vi "Start Scan.vi"(8 "error in (no error)":errorcluster, 10 "Init work":bool, 11 "Keithley 622x2182 Driver in":refnum<class "Keithley 622x2182 Driver.lvclass">) -> (0 "error out":errorcluster, 3 "Keithley 622x2182 Driver out":refnum<class "Keithley 622x2182 Driver.lvclass">)   [LabVIEW 2021, in "Keithley 622x2182 Driver.lvclass"]
uses:
  Keithley 622x2182 Driver.lvclass
  C:/GitHub/NHMFL_Core/Libraries/Instruments/VISA Instrument/VISA Instrument.lvclass
  VISA Instrument/VISA Instrument.lvclass/VISA Instrument.ctl
  VISA Instrument/Read VISA resource.vi
  VISA Instrument/Write VISA resource.vi
  Keithley 622x2182 Driver.lvclass/Keithley 622x2182 Driver.ctl
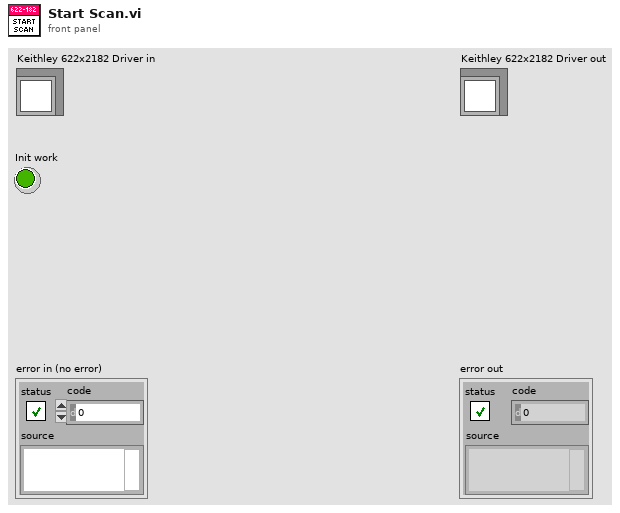
[diagram p1: front panel]
types:
  T1 = enum16{"Delta", "Diff. conductance", "Pulse delta sweep"}
  T2 = typedef "Stepper Config.ctl" = cluster{"Start":dbl, "End":dbl, "Step":dbl, "Delta":dbl, "Scan shape":enum16{"Sawtooth", "Triangular"}, "Append measurements":string[], "Pulse width":dbl, "Pulse interval":dbl, "Scan mode":enum16{"Delta", "Diff. conductance", "Pulse delta sweep"}}
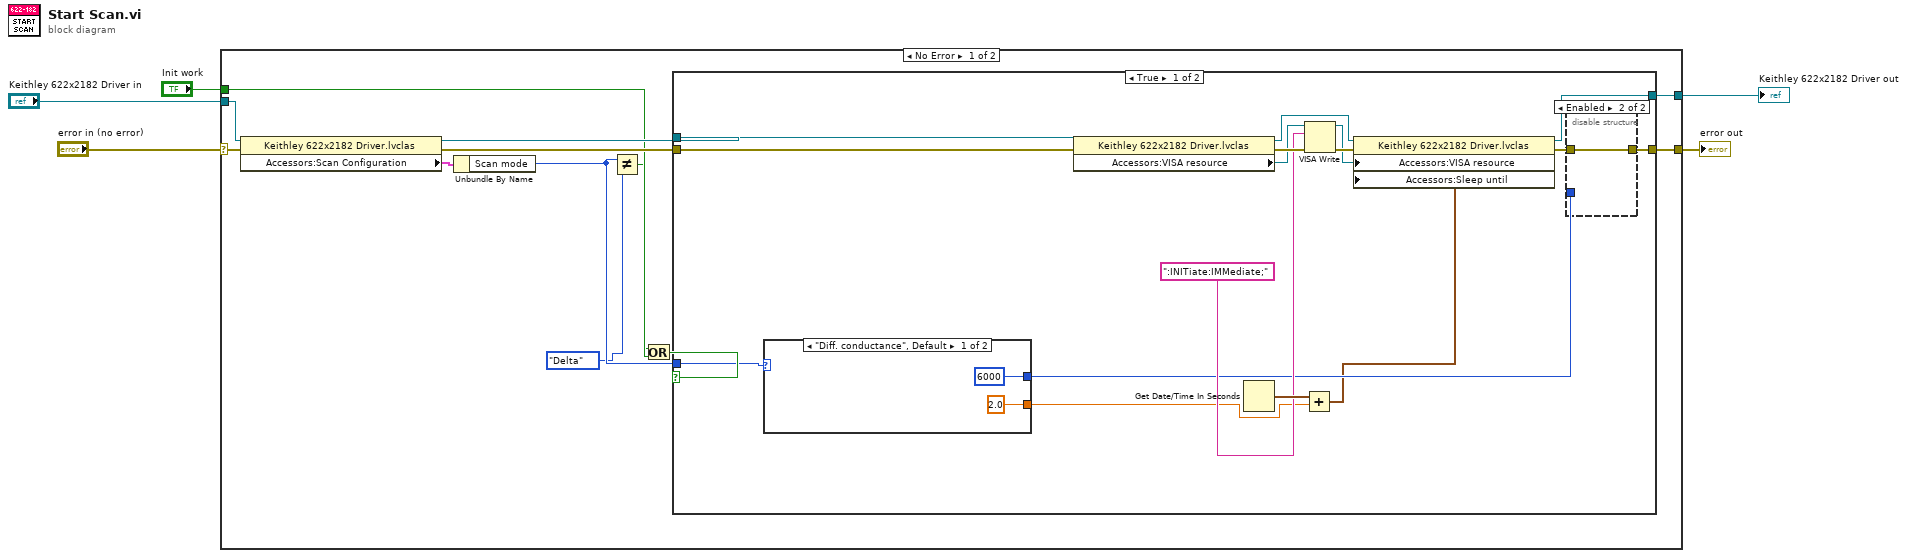
[diagram p0: block diagram]
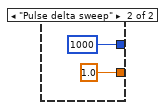
[diagram p2: hidden frame]
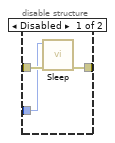
[diagram p3: hidden frame]
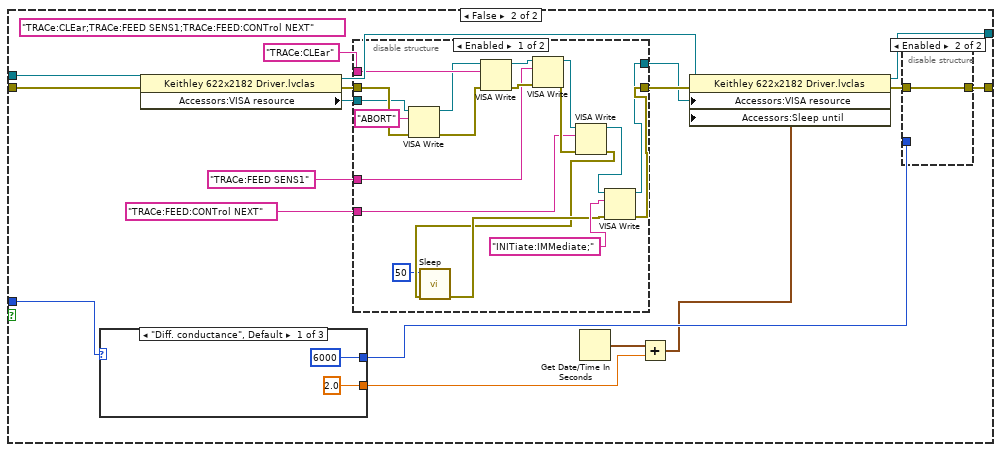
[diagram p4: hidden frame]
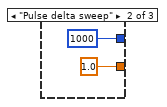
[diagram p6: hidden frame]
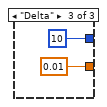
[diagram p7: hidden frame]
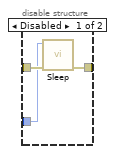
[diagram p8: hidden frame]
diagram:
  n1 = case shown="No Error" "error in (no error)" {
    selector: "error in (no error)" -> [w17 w92]
    tunnel: [w15 w92] -> w4
    tunnel: [w16 w91] -> w2
    tunnel: "Keithley 622x2182 Driver in" -> [w13 w91]
    tunnel: "Init work" -> [w8 _]
    frame No Error {
      n2 = property class="Keithley 622x2182 Driver.lvclas"(reference=w13, error in=w17) -> (reference out=w12:refnum<class "Keithley 622x2182 Driver.lvclass">, error out=w14:errorcluster, "Accessors:Scan Configuration"=w11:T2)
      n3 = Unbundle By Name(w11) -> ("Scan mode"=w10:T1)
      n4 = Not Equal?(x=w10, y=T1."Delta" ("Scan mode")) -> (x != y?=w7:bool)
      n5 = Or(x=w7, y=w8) -> (x .or. y?=w6:bool)
      n6 = case shown="True" w6 {
        tunnel: [w32 w58] -> w16
        tunnel: [w25 w51] -> w15
        tunnel: w10 -> [w23 w49]
        tunnel: w14 -> [w19 w45]
        tunnel: w12 -> [w18 w44]
        frame True {
          n7 = case shown="\"Diff. conductance\", Default" w23 {
            tunnel: [u32 6000 ("milliseconds to wait") u32 1000 ("milliseconds to wait")] -> w22
            tunnel: [2.0 ("y") 1.0 ("y")] -> w20
            frame "Diff. conductance", Default {
            }
            frame "Pulse delta sweep" {
            }
          }
          n8 = property class="Keithley 622x2182 Driver.lvclas"(reference=w18, error in=w19) -> (reference out=w33:refnum<class "Keithley 622x2182 Driver.lvclass">, error out=w30:errorcluster, "Accessors:VISA resource"=w27:refnum<visa-resource-name>)
          n9 = Get Date/Time In Seconds() -> (seconds since 1Jan1904=w31:timestamp)
          n10 = Add(x=w31, y=w20) -> (x+y=w21:timestamp)
          n11 = VISA Write(VISA resource name=w27, write buffer=":INITiate:IMMediate;", error in (no error)=w30) -> (VISA resource name out=w28:refnum<visa-resource-name>, error out=w29:errorcluster)  [unwired: 1 out]
          n12 = property class="Keithley 622x2182 Driver.lvclas"(reference=w33, error in=w29, "Accessors:VISA resource"=w28, "Accessors:Sleep until"=w21) -> (reference out=w32:refnum<class "Keithley 622x2182 Driver.lvclass">, error out=w24:errorcluster)
          n13 = disable-structure shown="Enabled" {
            disable-tunnel: [w40 w41] -> w25
            disable-tunnel: w24 -> [w39 w41]
            disable-tunnel: w22 -> [w38 _]
            frame Disabled {
              n14 = call "Sleep.vi"("error in"=w39, "milliseconds to wait"=w38) -> ("error out"=w40:errorcluster)  [unwired: 9 in]
            }
            frame Enabled {
            }
          }
        }
        frame False {
          (unwired) "TRACe:CLEar;TRACe:FEED SENS1;TRACe:FEED:CONTrol NEXT" ("write buffer")
          n15 = case shown="\"Diff. conductance\", Default" w49 {
            tunnel: [u32 6000 ("milliseconds to wait") u32 1000 ("milliseconds to wait") u32 10 ("milliseconds to wait")] -> w48
            tunnel: [2.0 ("y") 1.0 ("y") 0.01 ("y")] -> w46
            frame "Diff. conductance", Default {
            }
            frame "Pulse delta sweep" {
            }
            frame "Delta" {
            }
          }
          n16 = property class="Keithley 622x2182 Driver.lvclas"(reference=w44, error in=w45) -> (reference out=w59:refnum<class "Keithley 622x2182 Driver.lvclass">, error out=w56:errorcluster, "Accessors:VISA resource"=w53:refnum<visa-resource-name>)
          n17 = disable-structure shown="Enabled" {
            disable-tunnel: w56 -> [w66 w79]
            disable-tunnel: [w71 w79] -> w55
            disable-tunnel: [w69 w80] -> w54
            disable-tunnel: w53 -> [w64 w80]
            disable-tunnel: "TRACe:CLEar" ("write buffer") -> [w78 _]
            disable-tunnel: "TRACe:FEED SENS1" ("write buffer") -> [w75 _]
            disable-tunnel: "TRACe:FEED:CONTrol NEXT" ("write buffer") -> [w72 _]
            frame Enabled {
              n18 = VISA Write(VISA resource name=w64, write buffer="ABORT", error in (no error)=w66) -> (VISA resource name out=w65:refnum<visa-resource-name>, error out=w67:errorcluster)  [unwired: 1 out]
              n19 = VISA Write(VISA resource name=w65, write buffer=w78, error in (no error)=w67) -> (VISA resource name out=w76:refnum<visa-resource-name>, error out=w77:errorcluster)  [unwired: 1 out]
              n20 = VISA Write(VISA resource name=w76, write buffer=w75, error in (no error)=w77) -> (VISA resource name out=w74:refnum<visa-resource-name>, error out=w73:errorcluster)  [unwired: 1 out]
              n21 = VISA Write(VISA resource name=w74, write buffer=w72, error in (no error)=w73) -> (VISA resource name out=w70:refnum<visa-resource-name>, error out=w61:errorcluster)  [unwired: 1 out]
              n22 = call "Sleep.vi"("error in"=w61, "milliseconds to wait"=u32 50) -> ("error out"=w62:errorcluster)  [unwired: 9 in]
              n23 = VISA Write(VISA resource name=w70, write buffer="INITiate:IMMediate;", error in (no error)=w62) -> (VISA resource name out=w69:refnum<visa-resource-name>, error out=w71:errorcluster)  [unwired: 1 out]
            }
            frame Disabled {
            }
          }
          n24 = Get Date/Time In Seconds() -> (seconds since 1Jan1904=w57:timestamp)
          n25 = Add(x=w57, y=w46) -> (x+y=w47:timestamp)
          n26 = property class="Keithley 622x2182 Driver.lvclas"(reference=w59, error in=w55, "Accessors:VISA resource"=w54, "Accessors:Sleep until"=w47) -> (reference out=w58:refnum<class "Keithley 622x2182 Driver.lvclass">, error out=w50:errorcluster)
          n27 = disable-structure shown="Enabled" {
            disable-tunnel: [w89 w90] -> w51
            disable-tunnel: w50 -> [w88 w90]
            disable-tunnel: w48 -> [w87 _]
            frame Disabled {
              n28 = call "Sleep.vi"("error in"=w88, "milliseconds to wait"=w87) -> ("error out"=w89:errorcluster)  [unwired: 9 in]
            }
            frame Enabled {
            }
          }
        }
      }
    }
    frame Error {
    }
  }
  "error out" <- w4
  "Keithley 622x2182 Driver out" <- w2
